vi "Initialize.vi"(7 "Serial Configuration":cluster{"Baud Rate":u32}={"Baud Rate"=9600} {"Baud Rate" items=["300"=300, "600"=600, "1200"=1200, "2400"=2400, "4800"=4800, "9600"=9600, "19200"=19200]}, 8 "error in (no error)":errorcluster, 9 "Reset (True)":bool=TRUE, 10 "ID Query (True)":bool=TRUE, 11 "VISA resource name":refnum<visa-resource-name>) -> (0 "error out":errorcluster, 3 "VISA resource name out":refnum<visa-resource-name>)   [LabVIEW 2020, in "BK Precision 9200 Series.lvlib"]
doc: "Establishes communication with the instrument and optionally performs an instrument identification query and/or an instrument reset. It also places the instrument in a default state needed for other instrument driver operations. Therefore, call this VI before calling other instrument driver VIs for this instrument. Generally, you need to call the Initialize VI only once at the beginning of an application."
uses:
  BK Precision 9200 Series.lvlib
panel:
  # "(c) 2014 B&K Precision Corporation.  ALL RIGHTS RESERVED."
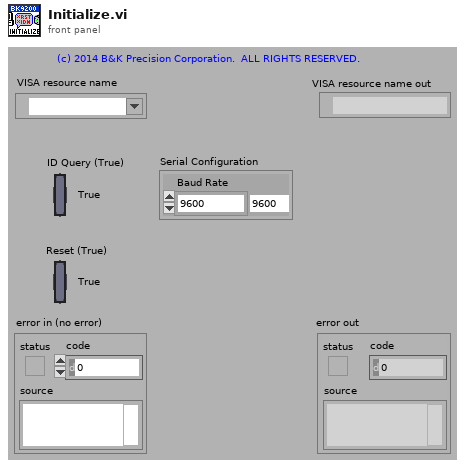
[diagram p1: front panel]
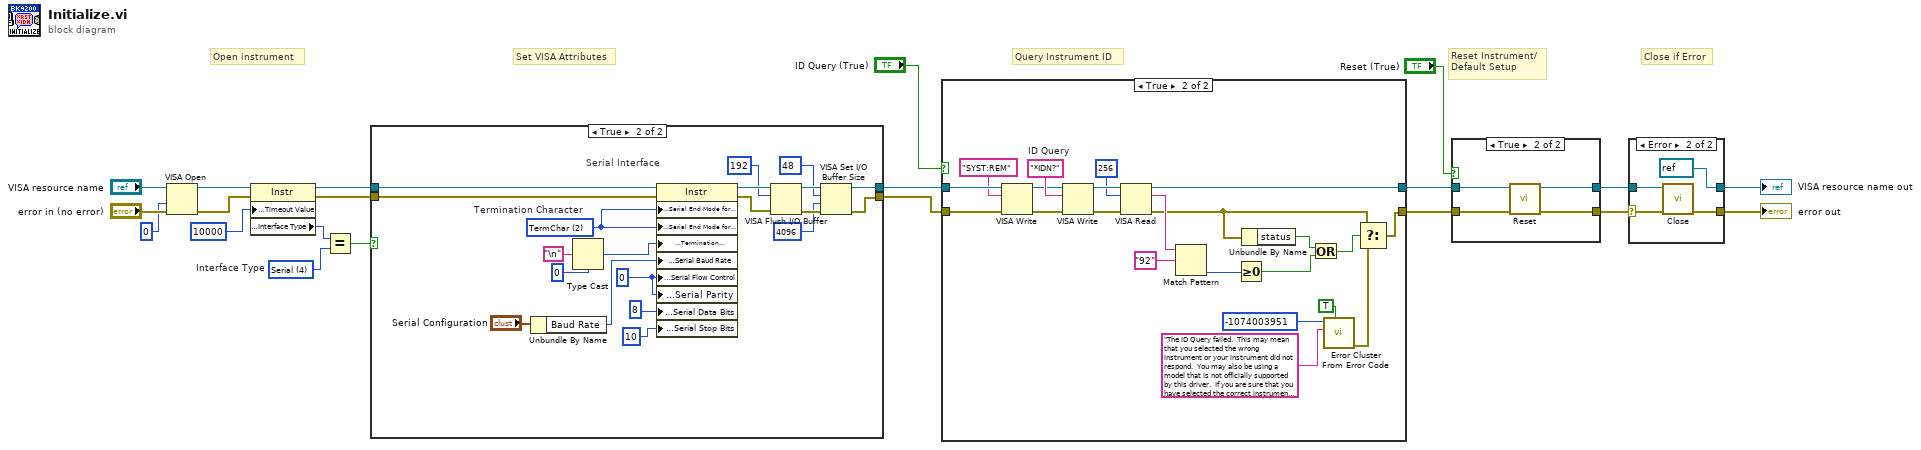
[diagram p0: block diagram]
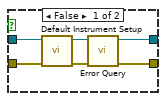
[diagram p4: hidden frame]
diagram:
  w8 = u16 4 items=["GPIB"=1, "Serial"=4, "TCPIP"=6]  # Interface Type
  # "Set VISA Attributes"
  # "Close if Error"
  # "Query Instrument ID"
  # "Reset Instrument/\nDefault Setup"
  # "Open instrument"
  n1 = VISA Open(access mode=u32 0, error in (no error)="error in (no error)", VISA resource name="VISA resource name") -> (VISA resource name=w2:refnum<visa-resource-name>, error out=w1:errorcluster)  [unwired: 2 in]
  n2 = property on="Property Node" class="Instr"(reference=w2, error in=w1, "General Settings:Timeout Value"=u32 10000) -> (reference out=w11:refnum<visa-resource-name>, error out=w10:errorcluster, "Interface Information:Interface Type"=w15:u16)
  n3 = Equal?(x=w15, y=w8) -> (x = y?=w9:bool)
  n4 = case shown="True" w9 {
    tunnel: [w23 w40] -> w13
    tunnel: [w22 w37] -> w12
    tunnel: w11 -> [w23 w42]
    tunnel: w10 -> [w22 w43]
    frame False {
      # "GPIB, USBTMC"
    }
    frame True {
      w28 = 0
      w30 = u16 2 items=["None", "LastBit", "TermChar"]  # Termination Character
      # "Serial Interface"
      n5 = Unbundle By Name("Serial Configuration") -> ("Baud Rate"=w24:u32)
      n6 = Type Cast(type=u8 0, x="\n" ("Line Feed Constant")) -> (*(type *) &x=w29:u8)
      n7 = property on="Property Node" class="Instr"(reference=w42, error in=w43, "Serial Settings:Serial End Mode for Reads"=w30, "Serial Settings:Serial End Mode for Writes"=w30, "Message Based Settings:Termination Character"=w29, "Serial Settings:Serial Baud Rate"=w24, "Serial Settings:Serial Flow Control"=w28, "Serial Settings:Serial Parity"=w28, "Serial Settings:Serial Data Bits"=8, "Serial Settings:Serial Stop Bits"=10) -> (reference out=w36:refnum<visa-resource-name>, error out=w39:errorcluster)
      n8 = VISA Flush I/O Buffer(VISA resource name=w36, mask (16)=u16 192, error in (no error)=w39) -> (VISA resource name out=w41:refnum<visa-resource-name>, error out=w38:errorcluster)
      n9 = VISA Set I/O Buffer Size(VISA resource name=w41, mask (16)=u16 48, size (4096)=u32 4096 ("size (0)"), error in (no error)=w38) -> (VISA resource name out=w40:refnum<visa-resource-name>, error out=w37:errorcluster)
    }
  }
  n10 = case shown="True" "ID Query (True)" {
    tunnel: [w44 w67] -> w20
    tunnel: [w45 w66] -> w21
    tunnel: w13 -> [w45 w48]
    tunnel: w12 -> [w44 w47]
    frame False {
    }
    frame True {
      w60 = "*IDN?"  # ID Query
      n11 = VISA Write(VISA resource name=w48, write buffer="SYST:REM", error in (no error)=w47) -> (VISA resource name out=w49:refnum<visa-resource-name>, error out=w50:errorcluster)  [unwired: 1 out]
      n12 = VISA Write(VISA resource name=w49, write buffer=w60, error in (no error)=w50) -> (VISA resource name out=w64:refnum<visa-resource-name>, error out=w63:errorcluster)  [unwired: 1 out]
      n13 = VISA Read(VISA resource name=w64, byte count=u32 256, error in (no error)=w63) -> (VISA resource name out=w66:refnum<visa-resource-name>, read buffer=w65:string, error out=w54:errorcluster)  [unwired: 1 out]
      n14 = Match Pattern(string=w65, regular expression="92") -> (offset past match=w55:i32)  [unwired: 1 in, 3 out]
      n15 = Greater Or Equal To 0?(x=w55) -> (x >= 0?=w52:bool)
      n16 = Unbundle By Name(w54) -> ("status"=w53:bool)
      n17 = Or(x=w53, y=w52) -> (x .or. y?=w51:bool)
      n18 = call <vilib>:"Error Cluster From Error Code.vi"("show call chain? (False)"=TRUE, "error message (\"\")"="The ID Query failed.  This may mean that you selected the wrong instrument or your instrument did not respond.  You may also be using a model that is not officially supported by this driver.  If you are sure that you have selected the correct instrument and it is responding, try disabling the ID Query." ("Source (VI Name)"), "error code (0)"=-1074003951 ("Code")) -> ("error out"=w59:errorcluster)  [unwired: 6 in]
      n19 = Select(t=w54, s=w51, f=w59) -> (s? t:f=w67:errorcluster)
    }
  }
  n20 = case shown="True" "Reset (True)" {
    tunnel: w20 -> [w72 w74]
    tunnel: [w69 w77] -> w3
    tunnel: w21 -> [w73 w75]
    tunnel: [w70 w76] -> w4
    frame False {
      n21 = call "Default Instrument Setup.vi"("error in (no error)"=w72, "VISA resource name"=w73) -> ("error out"=w68:errorcluster, "VISA resource name out"=w71:refnum<visa-resource-name>)  [unwired: 8 in]
      n22 = call "Error Query.vi"("error in (no error)"=w68, "VISA resource name"=w71) -> ("error out"=w69:errorcluster, "VISA resource name out"=w70:refnum<visa-resource-name>)  [unwired: 6 in, 2 out]
    }
    frame True {
      n23 = call "Reset.vi"("error in (no error)"=w74, "VISA resource name"=w75) -> ("error out"=w77:errorcluster, "VISA resource name out"=w76:refnum<visa-resource-name>)  [unwired: 8 in]
    }
  }
  n24 = case shown="Error" w3 {
    selector: w3 -> [w78 w81]
    tunnel: w4 -> [w79 w82]
    tunnel: [w79 refnum<visa-resource-name> refnum ("VISA resource name out")] -> w6
    tunnel: [w78 w83] -> w5
    frame No Error {
    }
    frame Error {
      n25 = call "Close.vi"("error in (no error)"=w81, "VISA resource name"=w82) -> ("error out"=w83:errorcluster)  [unwired: 9 in]
    }
  }
  "VISA resource name out" <- w6
  "error out" <- w5
